vi "颜色梯度.vi"() -> ()   [LabVIEW 2010]
panel:
  out "强度图表":dbl[][](graph)
  in  "旋钮":dbl(knob) scale=0.0..10.0
  out "量表":dbl(knob) scale=0.0..10.0
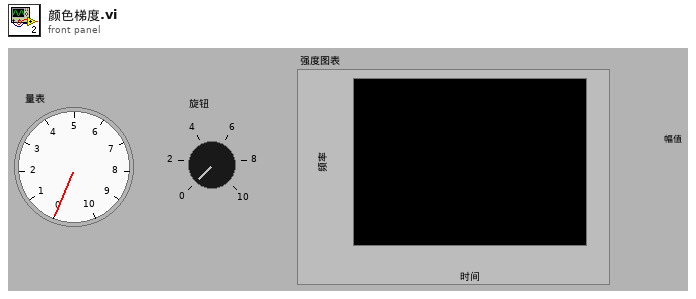
[diagram p1: front panel]
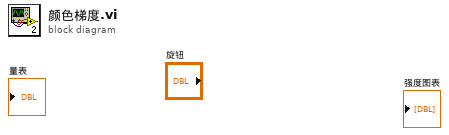
[diagram p0: block diagram]
diagram:
